vi "Framework Test.vi"() -> ()   [LabVIEW 2017]
uses:
  Source/DSF Configuration API/1.0.0/Public/Controls/DSF Direction.ctl
  Source/DSF Configuration API/1.0.0/Public/Controls/DSF Timing Info.ctl
  Built/Engine/DSF.Engine.lvlibp/DSF Configuration API/1.0.0/Public/Controls/DSF Settings Info.ctl
  Built/Engine/DSF.Engine.lvlibp/DSF Configuration API/1.0.0/Public/Controls/DSF Data Type.ctl
  <vilib>/Platform/TimedLoop/XDataNode/timing_clust.ctl
  <vilib>/Platform/TimedLoop/XDataNode/nitl_modes.ctl
  <vilib>/Platform/TimedLoop/XDataNode/wakeup.ctl
  Built/Engine/DSF.Engine.lvlibp/Engine/Classes/Debug/DSF.Engine.Debug Flags.FIFO.lvclass
  Built/Engine/DSF.Engine.lvlibp/Engine/Classes/Debug/DSF.Engine.Debug Flags.lvclass
  Built/Engine/DSF.Engine.lvlibp/Engine/Classes/Framework/DSF.Engine.Framework.lvclass
  <vilib>/National Instruments/Memory Manager/Classes/Pointer/Memory.Pointer.lvclass/Memory.Pointer.ctl
  <vilib>/National Instruments/Memory Manager/Classes/Pointer/Memory.Pointer.New.4B.vi
  <vilib>/National Instruments/Memory Manager/Classes/Pointer/Memory.Pointer.Write.0D.U32.vi
  <vilib>/National Instruments/Memory Manager/Classes/Pointer/Memory.Pointer.New.1B.vi
  <vilib>/National Instruments/Memory Manager/Classes/Pointer/Memory.Pointer.Write.0D.Bool.vi
  <vilib>/National Instruments/Memory Manager/Classes/Pointer/Memory.Pointer.Read.0D.I32.vi
  <vilib>/National Instruments/Memory Manager/Classes/Pointer/Memory.Pointer.Read.0D.U32.vi
  <vilib>/National Instruments/Memory Manager/Classes/Pointer/Memory.Pointer.Write.0D.I32.vi
  <vilib>/National Instruments/Memory Manager/Classes/Pointer/Memory.Pointer.Read.0D.Bool.vi
  <vilib>/National Instruments/Memory Manager/Classes/Pointer/Memory.Pointer.Allocate.vi
  <vilib>/National Instruments/Memory Manager/Classes/Pointer/Memory.Pointer.Write.No Check.0D.U32.vi
  <vilib>/National Instruments/Memory Manager/Classes/Pointer/Memory.Pointer.Parameter Check.Null Pointer.vi
  <vilib>/National Instruments/Memory Manager/Classes/Pointer/Memory.Pointer.Parameter Check.Subset.vi
  <vilib>/National Instruments/Memory Manager/Classes/Pointer/Memory.Pointer.Write.No Check.0D.Bool.vi
  <vilib>/National Instruments/Memory Manager/Classes/Pointer/Memory.Pointer.Read.No Check.0D.I32.vi
  <vilib>/National Instruments/Memory Manager/Classes/Pointer/Memory.Pointer.Read.No Check.0D.U32.vi
  <vilib>/National Instruments/Memory Manager/Classes/Pointer/Memory.Pointer.Write.No Check.0D.I32.vi
  <vilib>/National Instruments/Memory Manager/Classes/Pointer/Memory.Pointer.Read.No Check.0D.Bool.vi
  <vilib>/National Instruments/Memory Manager/Classes/Pointer/Memory.Pointer.Set Address.vi
  <vilib>/National Instruments/Memory Manager/Classes/Pointer/Memory.Pointer.Set Size.vi
  <vilib>/National Instruments/Memory Manager/Classes/Pointer/Memory.Pointer.Set Allocated.vi
  <vilib>/National Instruments/Memory Manager/Classes/Pointer/Memory.Pointer.Get Address.vi
  <vilib>/National Instruments/Memory Manager/Classes/Pointer/Memory.Pointer.Errors.vi
  <vilib>/National Instruments/Memory Manager/Classes/Pointer/Memory.Pointer.Errors.Null Pointer.vi
  <vilib>/National Instruments/Memory Manager/Classes/Pointer/Memory.Pointer.Errors.Out of Bounds.vi
  <vilib>/National Instruments/Memory Manager/Classes/Pointer/Memory.Pointer.Get Size.vi
  <vilib>/National Instruments/Memory Manager/Classes/Pointer/Memory.Pointer.Errors.Create Error.vi
  <vilib>/NI/Static Error Handling/VIs/Static Error Handling.Source Buffer.Write.String.vi
  <vilib>/National Instruments/Memory Manager/Classes/Pointer/Memory.Pointer.Errors.Write Pointer Size.vi
  <vilib>/NI/Static Error Handling/VIs/Static Error Handling.Source Buffer.Write.Numeric.Scalar.Base10.vi
  <vilib>/NI/Static Error Handling/VIs/Static Error Handling.Source Buffer.Write.Numeric.Scalar.Base10 (U64).vi
  <vilib>/NI/Static Error Handling/VIs/Static Error Handling.Error Cluster Constant.vi
  <vilib>/NI/Static Error Handling/VIs/Static Error Handling.Error Cluster Constant (512B).vi
  <vilib>/NI/Static Error Handling/VIs/Static Error Handling.Parameters.Status.Set.vi
  <vilib>/NI/Static Error Handling/VIs/Static Error Handling.Parameters.Code.Set.vi
  <vilib>/NI/Static Error Handling/VIs/Static Error Handling.Parameters.VI Source.Set.vi
  <vilib>/National Instruments/Memory Manager/Constants/Memory.Constants.vi
  <vilib>/National Instruments/Memory Manager/Constants/Memory.Constants.Library Name.vi
  <vilib>/National Instruments/Memory Manager/Classes/Pointer/Memory.Pointer.Errors.Get Info.vi
  <vilib>/National Instruments/Memory Manager/Classes/Pointer/Memory.Pointer.lvclass
  <vilib>/platform/TimedLoop/XDataNode/XDataNode.xnode
  <vilib>/Platform/TimedLoop/XDataNode/XDNodeRunTimeDep.lvlib
  Built/Engine/DSF.Engine.lvlibp/Shared/Classes/Framework/DSF.Shared.Configuration.Framework.lvclass
  Built/Engine/DSF.Engine.lvlibp/Engine/Classes/Pointer/DSF.Engine.Pointer.DBL.lvclass
  Built/Engine/DSF.Engine.lvlibp/Engine/Classes/Status/DSF.Engine.Status.Framework.lvclass
  Built/Engine/DSF.Engine.lvlibp/Engine/Classes/Status/DSF.Engine.Status.Framework.Performance.lvclass
  C:/Git/DSF/DSF Core/Built/Engine/DSF.Engine.lvlibp/1abvi3w/vi.lib/National Instruments/Memory Manager/Classes/Pointer/Memory.Pointer.lvclass
  Source/DSF Configuration API/1.0.0/DSF Configuration API.lvlib
  Built/Engine/DSF.Engine.lvlibp/DSF Configuration API/1.0.0/DSF Configuration API.lvlib
panel:
  in  "Plugins":T5(array[cluster])=[{"plugin class"="DSF.Transceiver.UDP", "group configs"=[{"direction"=enum."Tx", "timing"={"priority"=100, "decimation"=1, "offset"=0}, "settings"=[], "transfer configs"=[{"random types?"=FALSE, "non-random type"=enum."DBL", "channel count"=100, "settings"=[{"key"="Destination Address", "value"="localhost"}, {"key"="Destination Port", "value"="60000"}]}]}, {"direction"=enum."Tx", "timing"={"priority"=100, "decimation"=2, "offset"=0}, "settings"=[], "transfer configs"=[{"random types?"=FALSE, "non-random type"=enum."DBL", "channel count"=100, "settings"=[{"key"="Destination Address", "value"="localhost"}, {"key"="Destination Port", "value"="60001"}]}]}, {"direction"=enum."Tx", "timing"={"priority"=100, "decimation"=3, "offset"=0}, "settings"=[], "transfer configs"=[{"random types?"=FALSE, "non-random type"=enum."DBL", "channel count"=100, "settings"=[{"key"="Destination Address", "value"="localhost"}, {"key"="Destination Port", "value"="60002"}]}]}, {"direction"=enum."Tx", "timing"={"priority"=100, "decimation"=4, "offset"=0}, "settings"=[], "transfer configs"=[{"random types?"=FALSE, "non-random type"=enum."DBL", "channel count"=100, "settings"=[{"key"="Destination Address", "value"="localhost"}, {"key"="Destination Port", "value"="60003"}]}]}], "plugin timing"={"priority"=100, "decimation"=1, "offset"=0}, "settings"=[{"key"="Local Port", "value"="50000"}]}]
  in  "infinite timeouts":bool
  out "Framework Error":errorcluster
  out "Tx duration":u32 format="%d us"
  out "Rx duration":u32 format="%d us"
  out "Actual PCL Frequency":dbl format="%.0pHz"
  in  "Transceiver Count":i32=4
  in  "Configuration Path":path=path "C:/Users/Admin/Desktop/test.json"
  out "Framework Iteration":i32 format="%d cycles"
  out "Actual Period":u32 format="%d us"
  in  "Target PCL Frequency":dbl=100.0 caption="Target Period" format="%.0pHz"
  in  "stop":bool
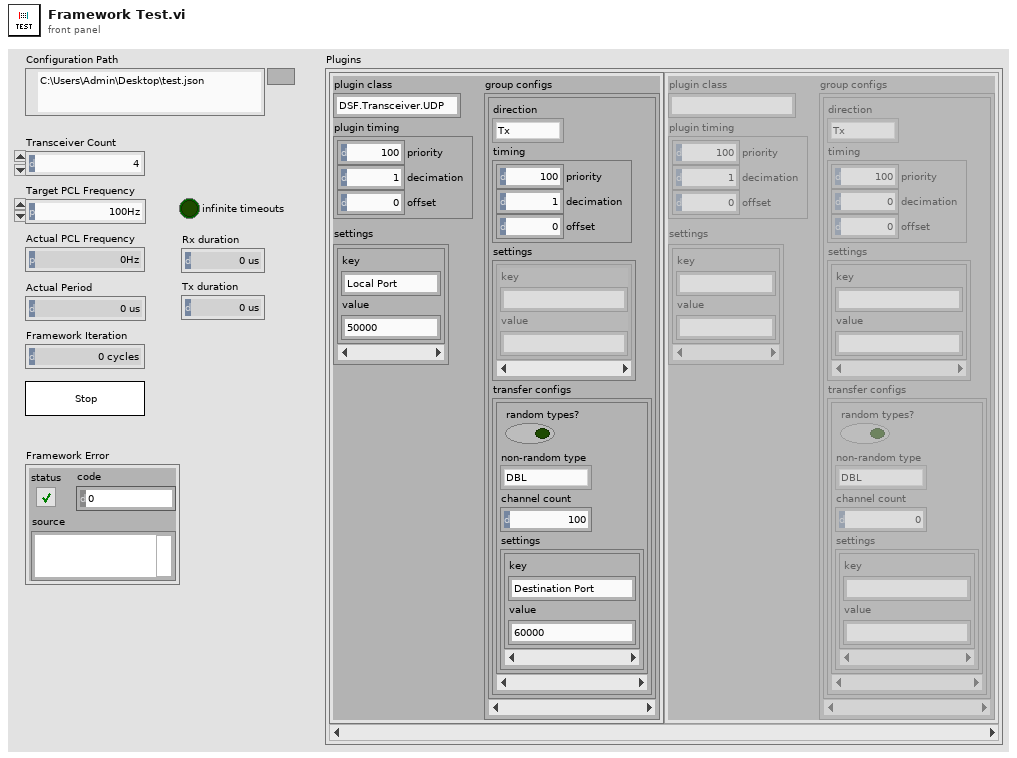
[diagram p1: front panel]
types:
  T1 = typedef "DSF Configuration API.lvlib/DSF Direction.ctl" = enum8{"Tx", "Rx"}
  T2 = typedef "DSF Configuration API.lvlib/DSF Timing Info.ctl" = cluster{"priority":u64, "decimation":u64, "offset":u64}
  T3 = typedef "DSF.Engine.lvlibp/DSF Configuration API.lvlib/DSF Settings Info.ctl" = cluster{"key":string, "value":string}[]
  T4 = typedef "DSF.Engine.lvlibp/DSF Configuration API.lvlib/DSF Data Type.ctl" = enum8{"Bool", "SGL", "DBL", "I8", "I16", "I32", "I64", "U8", "U16", "U32", "U64"}
  T5 = cluster{"plugin class":string, "group configs":cluster{"direction":T1, "timing":T2, "settings":T3, "transfer configs":cluster{"random types?":bool, "non-random type":T4, "channel count":i32, "settings":T3}[]}[], "plugin timing":T2, "settings":T3}[]
  T6 = typedef "DSF.Engine.lvlibp/DSF Configuration API.lvlib/DSF Engine Framework Configuration.ctl" = cluster{"Plugins":T7[]}
  T7 = typedef "DSF.Engine.lvlibp/DSF Configuration API.lvlib/DSF Engine Plugin Configuration.ctl" = cluster{"name":string, "class":string, "cycle timing":T8, "Transfer Groups":T9[], "settings":T3}
  T8 = typedef "DSF.Engine.lvlibp/DSF Configuration API.lvlib/DSF Timing Info.ctl" = cluster{"priority":u64, "decimation":u64, "offset":u64}
  T9 = typedef "DSF.Engine.lvlibp/DSF Configuration API.lvlib/DSF Engine Transfer Group Configuration.ctl" = cluster{"name":string, "direction":T10, "cycle timing":T8, "Transfers":T11[], "settings":T3}
  T10 = typedef "DSF.Engine.lvlibp/DSF Configuration API.lvlib/DSF Direction.ctl" = enum8{"Tx", "Rx"}
  T11 = typedef "DSF.Engine.lvlibp/DSF Configuration API.lvlib/DSF Engine Transfer Configuration.ctl" = cluster{"name":string, "byte order":T12, "channel configurations":T13[], "settings":T3}
  T12 = typedef "DSF.Engine.lvlibp/DSF Configuration API.lvlib/DSF Byte Order.ctl" = enum8{"big-endian", "little-endian"}
  T13 = typedef "DSF.Engine.lvlibp/DSF Configuration API.lvlib/DSF Engine Channel Configuration.ctl" = cluster{"engine offset":u64, "name":string, "data type":T4, "count":u64, "buffer offset":u64, "settings":T3}
  T14 = typedef "XDNodeRunTimeDep.lvlib/timing_clust.ctl" = cluster{"Expected End [f-1]":u64, "Actual End [f-1]":u64, "Finished Late? [f-1]":bool, "Expected End [i-1]":u64, "Actual End [i-1]":u64, "Finished Late? [i-1]":bool, "Expected Start [i]":u64, "Actual Start [i]":u64, "Expected Start [f]":u64, "Actual Start [f]":u64, "Source Name":string, "Structure Name":string, "Period":i64, "Deadline":i64, "Offset":i64, "Start":i64, "Priority":i32, "Timeout":i32, "Mode":T15, "Wakeup Reason":T16, "Error":errorcluster, "Source Type":string, "Secondary Source Type":string, "Global End Time":u64, "Global Start Time":u64, "Frame Duration":u64, "Iteration Duration":u64, "Assigned CPU":i32, "I/O Scan Engine Mode":u32}
  T15 = typedef "XDNodeRunTimeDep.lvlib/nitl_modes.ctl" = enum32{"No Change", "Process missed periods, maintain original phase", "Discard missed periods, maintain original phase", "Process missed periods, ignore original phase", "Discard missed periods, ignore original phase"}
  T16 = typedef "XDNodeRunTimeDep.lvlib/wakeup.ctl" = enum32{"Normal", "Aborted", "Asynchronous wakeup", "Timing source error", "Timed loop error", "Timeout"}
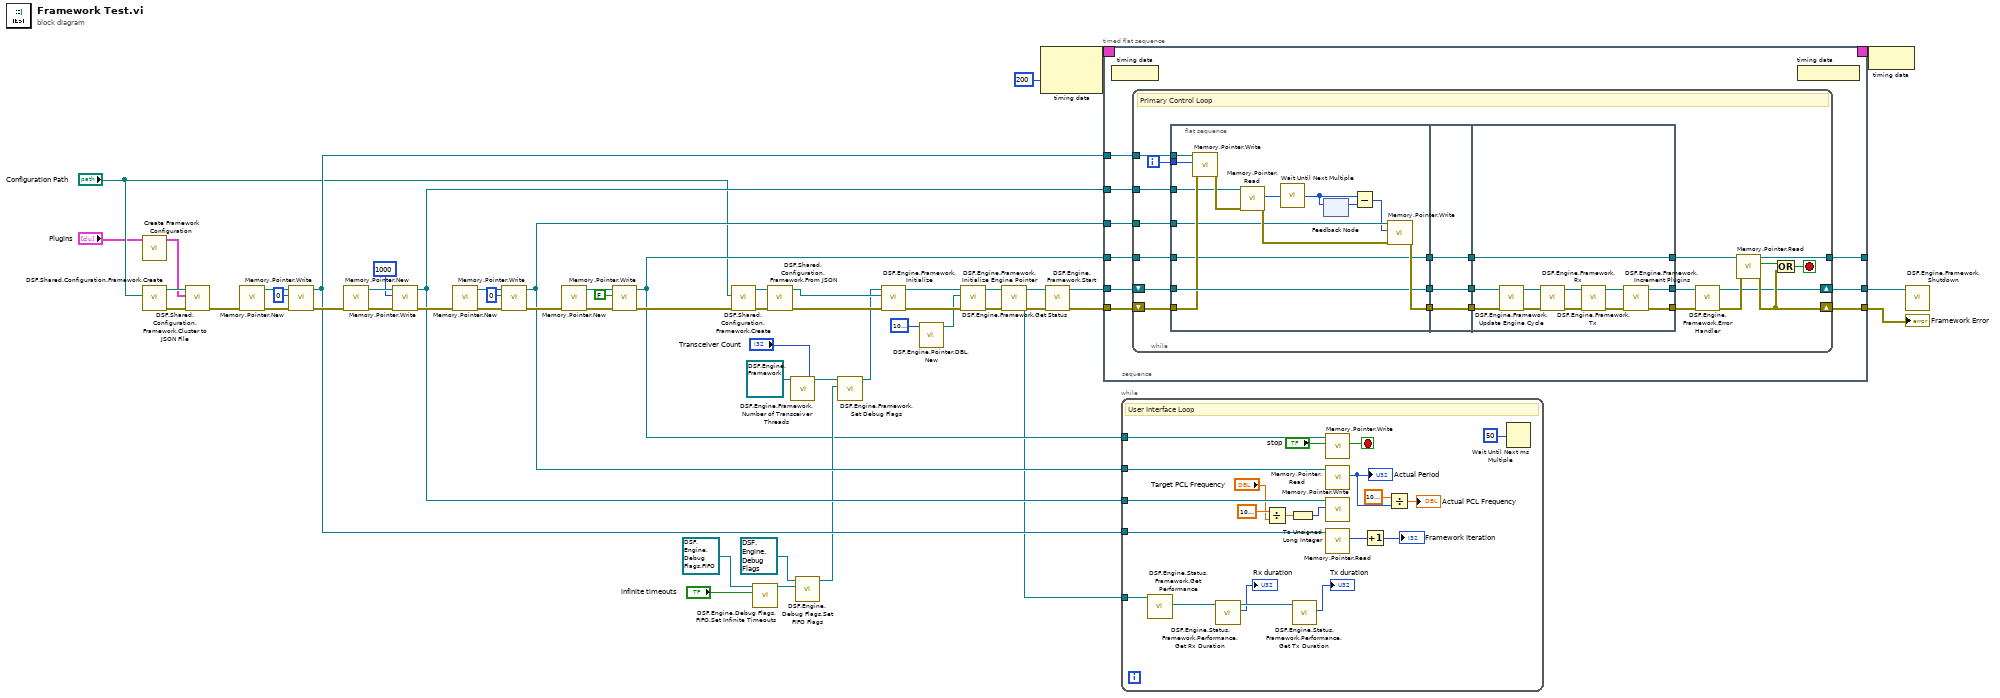
[diagram p0: block diagram]
diagram:
  n1 = call "Create Framework Configuration.vi"("Plugins"="Plugins") -> ("Framework Configuration"=w14:T6)  [unwired: 10 in]
  n2 = call "DSF.Shared.Configuration.Framework.Create.vi"("configuration path"="Configuration Path") -> ("error out"=w28:errorcluster, "Framework Configuration"=w29:refnum<class "DSF.Shared.Configuration.Framework.lvclass">)  [unwired: 9 in]
  n3 = call "DSF.Shared.Configuration.Framework.Cluster to JSON File.vi"("error in (no error)"=w28, "Framework Configuration"=w14, "Framework Configuration in"=w29) -> ("error out"=w27:errorcluster)  [unwired: 7 in, 1 out]
  n4 = call-poly <vilib>:"Memory.Pointer.New.vi"("error in (no error)"=w27) -> ("error out"=w35:errorcluster, "Pointer"=w36:refnum<class "Memory.Pointer.lvclass">)  [unwired: 9 in]
  n5 = call-poly <vilib>:"Memory.Pointer.Write.vi"("error in (no error)"=w35, "value"=u32 0, "Pointer in"=w36) -> ("error out"=w34:errorcluster, "Pointer out"=w31:refnum<class "Memory.Pointer.lvclass">)  [unwired: 5 in, 2 out]
  n6 = call-poly <vilib>:"Memory.Pointer.New.vi"("error in (no error)"=w34) -> ("error out"=w42:errorcluster, "Pointer"=w43:refnum<class "Memory.Pointer.lvclass">)  [unwired: 9 in]
  n7 = call-poly <vilib>:"Memory.Pointer.Write.vi"("error in (no error)"=w42, "value"=u32 1000, "Pointer in"=w43) -> ("error out"=w41:errorcluster, "Pointer out"=w37:refnum<class "Memory.Pointer.lvclass">)  [unwired: 5 in, 2 out]
  n8 = call-poly <vilib>:"Memory.Pointer.New.vi"("error in (no error)"=w41) -> ("error out"=w40:errorcluster, "Pointer"=w44:refnum<class "Memory.Pointer.lvclass">)  [unwired: 9 in]
  n9 = call-poly <vilib>:"Memory.Pointer.Write.vi"("error in (no error)"=w40, "value"=u32 0, "Pointer in"=w44) -> ("error out"=w39:errorcluster, "Pointer out"=w38:refnum<class "Memory.Pointer.lvclass">)  [unwired: 5 in, 2 out]
  n10 = call-poly <vilib>:"Memory.Pointer.New.vi"("error in (no error)"=w39) -> ("error out"=w47:errorcluster, "Pointer"=w46:refnum<class "Memory.Pointer.lvclass">)  [unwired: 9 in]
  n11 = call-poly <vilib>:"Memory.Pointer.Write.vi"("error in (no error)"=w47, "value"=FALSE, "Pointer in"=w46) -> ("error out"=w30:errorcluster, "Pointer out"=w17:refnum<class "Memory.Pointer.lvclass">)  [unwired: 5 in, 2 out]
  n12 = call "DSF.Shared.Configuration.Framework.Create.vi"("error in (no error)"=w30, "configuration path"="Configuration Path") -> ("error out"=w32:errorcluster, "Framework Configuration"=w33:refnum<class "DSF.Shared.Configuration.Framework.lvclass">)  [unwired: 8 in]
  n13 = call "DSF.Engine.Debug Flags.FIFO.Set Infinite Timeouts.vi"("infinite timeouts"="infinite timeouts", "FIFO Debug Flags in"=refnum<class "DSF.Engine.Debug Flags.FIFO.lvclass"> refnum) -> ("FIFO Debug Flags out"=w22:refnum<class "DSF.Engine.Debug Flags.FIFO.lvclass">)  [unwired: 9 in]
  n14 = call "DSF.Shared.Configuration.Framework.From JSON.vi"("error in (no error)"=w32, "Framework Configuration in"=w33) -> ("error out"=w54:errorcluster, "Framework Configuration out"=w16:refnum<class "DSF.Shared.Configuration.Framework.lvclass">)  [unwired: 8 in]
  n15 = call "DSF.Engine.Framework.Number of Transceiver Threads.vi"("transceiver count"="Transceiver Count", "Framework in"=refnum<class "DSF.Engine.Framework.lvclass"> refnum) -> ("Framework out"=w23:refnum<class "DSF.Engine.Framework.lvclass">)  [unwired: 8 in, 1 out]
  n16 = call "DSF.Engine.Debug Flags.Set FIFO Flags.vi"("FIFO"=w22, "Debug Flags in"=refnum<class "DSF.Engine.Debug Flags.lvclass"> refnum) -> ("Debug Flags out"=w18:refnum<class "DSF.Engine.Debug Flags.lvclass">)  [unwired: 9 in]
  n17 = call "DSF.Engine.Framework.Set Debug Flags.vi"("Debug Flags"=w18, "Framework in"=w23) -> ("Framework out"=w4:refnum<class "DSF.Engine.Framework.lvclass">)  [unwired: 9 in]
  n18 = call "DSF.Engine.Framework.Initialize.vi"("error in (no error)"=w54, "Framework Configuration"=w16, "Framework type"=w4) -> ("error out"=w8:errorcluster, "Framework out"=w9:refnum<class "DSF.Engine.Framework.lvclass">)  [unwired: 7 in]
  n19 = call "DSF.Engine.Pointer.DBL.New.vi"("channel count"=u64 1000000) -> ("DBL Pointer out"=w3:refnum<class "DSF.Engine.Pointer.DBL.lvclass">)  [unwired: 9 in, 1 out]
  n20 = call "DSF.Engine.Framework.Initialize Engine Pointer.vi"("error in (no error)"=w8, "Engine Pointer"=w3, "Framework in"=w9) -> ("error out"=w5:errorcluster, "Framework out"=w7:refnum<class "DSF.Engine.Framework.lvclass">)  [unwired: 7 in]
  n21 = call "DSF.Engine.Framework.Get Status.vi"("Framework in"=w7) -> ("Status"=w2:refnum<class "DSF.Engine.Status.Framework.lvclass">, "Framework out"=w6:refnum<class "DSF.Engine.Framework.lvclass">)  [unwired: 9 in]
  n22 = node-c288(200 ("Priority")) -> (w49:T14)  [unwired: 1 in]
  n23 = call "DSF.Engine.Framework.Start.vi"("error in (no error)"=w5, "Framework in"=w6) -> ("error out"=w52:errorcluster, "Framework out"=w53:refnum<class "DSF.Engine.Framework.lvclass">)  [unwired: 8 in]
  n24 = timed-sequence {
    timing: w49 -> [_]
    timing-out: [_] -> w48
    tunnel: w53 -> [w63]
    tunnel: w52 -> [w62]
    tunnel: [w61] -> w51
    tunnel: [w60] -> w50
    tunnel: w17 -> [w59]
    tunnel: w37 -> [w58]
    tunnel: w38 -> [w57]
    tunnel: w31 -> [w56]
    tunnel: [w55] -> _
    n25 = timed-flat-sequence {
      tunnel: w63 -> [w72]
      tunnel: w62 -> [w71]
      tunnel: [w70] -> w61
      tunnel: [w69] -> w60
      tunnel: w59 -> [w68]
      tunnel: w58 -> [w67]
      tunnel: w57 -> [w66]
      tunnel: w56 -> [w65]
      tunnel: [w64] -> w55
      n26 = node-c288() -> ()  [unwired: 1 in]
      n27 = while {
        shift-right: [w73] -> w70
        shift-left: w72 -> [w93]
        shift-right: [w87] -> w69
        shift-left: w71 -> [w94]
        tunnel: w68 -> [w92]
        tunnel: w67 -> [w90]
        tunnel: w66 -> [w89]
        tunnel: w65 -> [w85]
        tunnel: [w77] -> w64
        i -> [w84]
        stop <- w86 stop-if-true
        # "Primary Control Loop"
        n28 = flat-sequence {
          tunnel: w94 -> [w103]
          tunnel: w93 -> [w106]
          tunnel: w92 -> [w99]
          tunnel: [w107] -> w83
          tunnel: [w106] -> w81
          tunnel: [w99] -> w79
          tunnel: w90 -> [w101]
          tunnel: w89 -> [w100]
          tunnel: w85 -> [w104]
          tunnel: w84 -> [w97]
          tunnel: w83 -> [w111]
          tunnel: [w111] -> w82
          tunnel: w81 -> [w110]
          tunnel: [w110] -> w80
          tunnel: w79 -> [w109]
          tunnel: [w109] -> w78
          tunnel: w82 -> [w114]
          tunnel: w80 -> [w115]
          tunnel: w78 -> [w116]
          tunnel: [w116] -> w91
          tunnel: [w118] -> w76
          tunnel: [w117] -> w75
          frame #0 {
            n29 = call-poly <vilib>:"Memory.Pointer.Write.vi"("error in (no error)"=w103, "value"=w97, "Pointer in"=w104) -> ("error out"=w102:errorcluster)  [unwired: 5 in, 3 out]
            n30 = call-poly <vilib>:"Memory.Pointer.Read.vi"("error in (no error)"=w102, "Pointer in"=w101) -> ("error out"=w105:errorcluster, "value out"=w96:u32)  [unwired: 6 in, 2 out]
            n31 = call "Wait Until Next Multiple"("Count(uSec)"=w96) -> ("Tick Count(uSec)"=w98:u32)
            n32 = feedback #1() -> (w108:u32)  [unwired: 1 in]
            n33 = feedback-in #1(w98) -> ()
            n34 = Subtract(x=w98, y=w108) -> (x-y=w95:u32)
            n35 = call-poly <vilib>:"Memory.Pointer.Write.vi"("error in (no error)"=w105, "value"=w95, "Pointer in"=w100) -> ("error out"=w107:errorcluster)  [unwired: 5 in, 3 out]
          }
          frame #1 {
          }
          frame #2 {
            n36 = call-dynamic "DSF.Engine.Framework.Update Engine Cycle.vi"("error in (no error)"=w114, "Framework in"=w115) -> ("error out"=w112:errorcluster, "Framework out"=w113:refnum<class "DSF.Engine.Framework.lvclass">)  [unwired: 8 in]
            n37 = call "DSF.Engine.Framework.Rx.vi"("error in (no error)"=w112, "Framework in"=w113) -> ("error out"=w122:errorcluster, "Framework out"=w121:refnum<class "DSF.Engine.Framework.lvclass">)  [unwired: 8 in]
            n38 = call "DSF.Engine.Framework.Tx.vi"("error in (no error)"=w122, "Framework in"=w121) -> ("error out"=w119:errorcluster, "Framework out"=w120:refnum<class "DSF.Engine.Framework.lvclass">)  [unwired: 8 in]
            n39 = call "DSF.Engine.Framework.Increment Plugins.vi"("error in (no error)"=w119, "Framework in"=w120) -> ("error out"=w117:errorcluster, "Framework out"=w118:refnum<class "DSF.Engine.Framework.lvclass">)  [unwired: 8 in]
          }
        }
        n40 = call "DSF.Engine.Framework.Error Handler.vi"("error in (no error)"=w75, "Framework in"=w76) -> ("error out"=w74:errorcluster, "Framework out"=w73:refnum<class "DSF.Engine.Framework.lvclass">)  [unwired: 8 in]
        n41 = call-poly <vilib>:"Memory.Pointer.Read.vi"("error in (no error)"=w74, "Pointer in"=w91) -> ("error out"=w87:errorcluster, "value out"=w88:bool, "Pointer out"=w77:refnum<class "Memory.Pointer.lvclass">)  [unwired: 6 in, 1 out]
        n42 = Or(x=w88, y=w87) -> (x .or. y?=w86:bool)
      }
      n43 = node-c288() -> ()  [unwired: 1 out]
    }
  }
  "Framework Error" <- w50
  n44 = while {
    tunnel: w17 -> [w144]
    tunnel: w38 -> [w140]
    tunnel: w37 -> [w141]
    tunnel: w31 -> [w134]
    tunnel: w2 -> [w132]
    stop <- w145 stop-if-true
    # "User Interface Loop"
    n45 = call "DSF.Engine.Status.Framework.Get Performance.vi"("Framework Status in"=w132) -> ("Framework Performance"=w131:refnum<class "DSF.Engine.Status.Framework.Performance.lvclass">)  [unwired: 9 in, 1 out]
    n46 = call "DSF.Engine.Status.Framework.Performance.Get Rx Duration.vi"("Framework Performance in"=w131) -> ("rx duration"=→"Rx duration":u32, "Framework Performance out"=w130:refnum<class "DSF.Engine.Status.Framework.Performance.lvclass">)  [unwired: 8 in, 1 out]
    n47 = Divide(x=1000000.0 ("y"), y="Target PCL Frequency") -> (x/y=w137:dbl)
    n48 = To Unsigned Long Integer(number=w137) -> (unsigned 32bit integer=w126:u32)
    n49 = call "DSF.Engine.Status.Framework.Performance.Get Tx Duration.vi"("Framework Performance in"=w130) -> ("tx duration"=→"Tx duration":u32)  [unwired: 8 in, 2 out]
    n50 = call-poly <vilib>:"Memory.Pointer.Write.vi"("value"="stop", "Pointer in"=w144) -> ("value"=w145:bool)  [unwired: 6 in, 3 out]
    n51 = call-poly <vilib>:"Memory.Pointer.Read.vi"("Pointer in"=w140) -> ("value out"=w127:u32)  [unwired: 7 in, 3 out]
    "Actual Period" <- w127
    n52 = call-poly <vilib>:"Memory.Pointer.Write.vi"("value"=w126, "Pointer in"=w141) -> ()  [unwired: 6 in, 4 out]
    n53 = call-poly <vilib>:"Memory.Pointer.Read.vi"("Pointer in"=w134) -> ("value out"=w125:i32)  [unwired: 7 in, 3 out]
    n54 = Increment(x=w125) -> (x+1=→"Framework Iteration":i32)
    n55 = Divide(x=1000000.0, y=w127) -> (x/y=→"Actual PCL Frequency":dbl)
    n56 = Wait Until Next ms Multiple(millisecond multiple=u32 50 ("milliseconds to wait")) -> ()  [unwired: 1 out]
  }
  n57 = node-c288(w48) -> ()
  n58 = call "DSF.Engine.Framework.Shutdown.vi"("Framework in"=w51) -> ()  [unwired: 9 in, 2 out]
